vi "Config GSM Framed Timeslot.vi"(0 "VISA Resource Name":refnum<visa-resource-name>, 1 "Data (0:PN9)":T1(ring), 2 "FIX4 (0000)":i16 format="%.0b", 3 "Extended Tail Bits (3A)":i32=58 format="%.0x", 4 "User File Name (BIN_DATA)":string="BIN_DATA", 5 "error in (no error)":errorcluster {"code" format="%.0x"}, 6 "Timeslot Type (1:NORMAL)":T2(ring)=enum."NORMAL", 7 "Synch Sequence (000)":string, 8 "Status (T:ON)":bool=TRUE, 9 "Training Sequence (0970897)":string="0970897", 10 "Timeslot (0)":i16, 11 "Steal Bit (0)":i8 format="%.0x") -> (14 "VISA Resource Name Out":refnum<visa-resource-name>, 19 "error out":errorcluster {"code" format="%.0x"})   [LabVIEW 2014, in "Agilent ESG Series.lvlib"]
doc: "This VI is used configure a specified Timeslot.\nRun the Config GSM Framed.vi before running this vi.\nRun this vi multiple times to configure multiple Timeslots."
uses:
  Agilent ESG Series.lvlib
panel:
  # "ON"
  # "OFF"
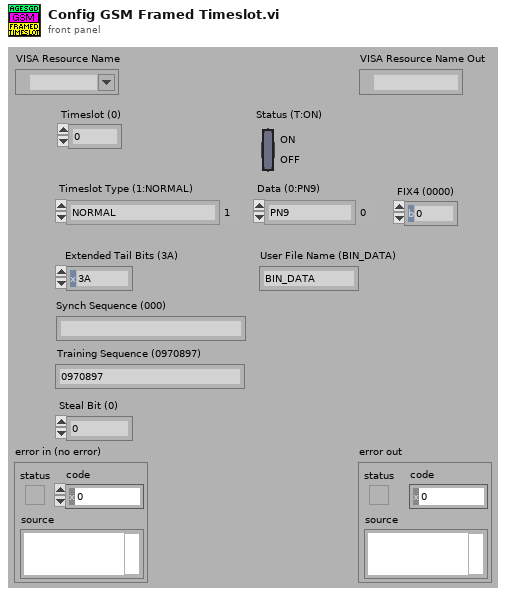
[diagram p1: front panel]
types:
  T1 = enum16{"PN9", "PN15", "FIX4", "USER FILE", "EXT", "4 1's & 4 0's", "8 1's & 8 0's", "16 1's & 16 0's", "32 1's & 32 0's", "64 1's & 64 0's"}
  T2 = enum16{"CUSTOM", "NORMAL", "FCORRECTION", "SYNC", "DUMMY", "ACCESS", "NORMAL ALL"}
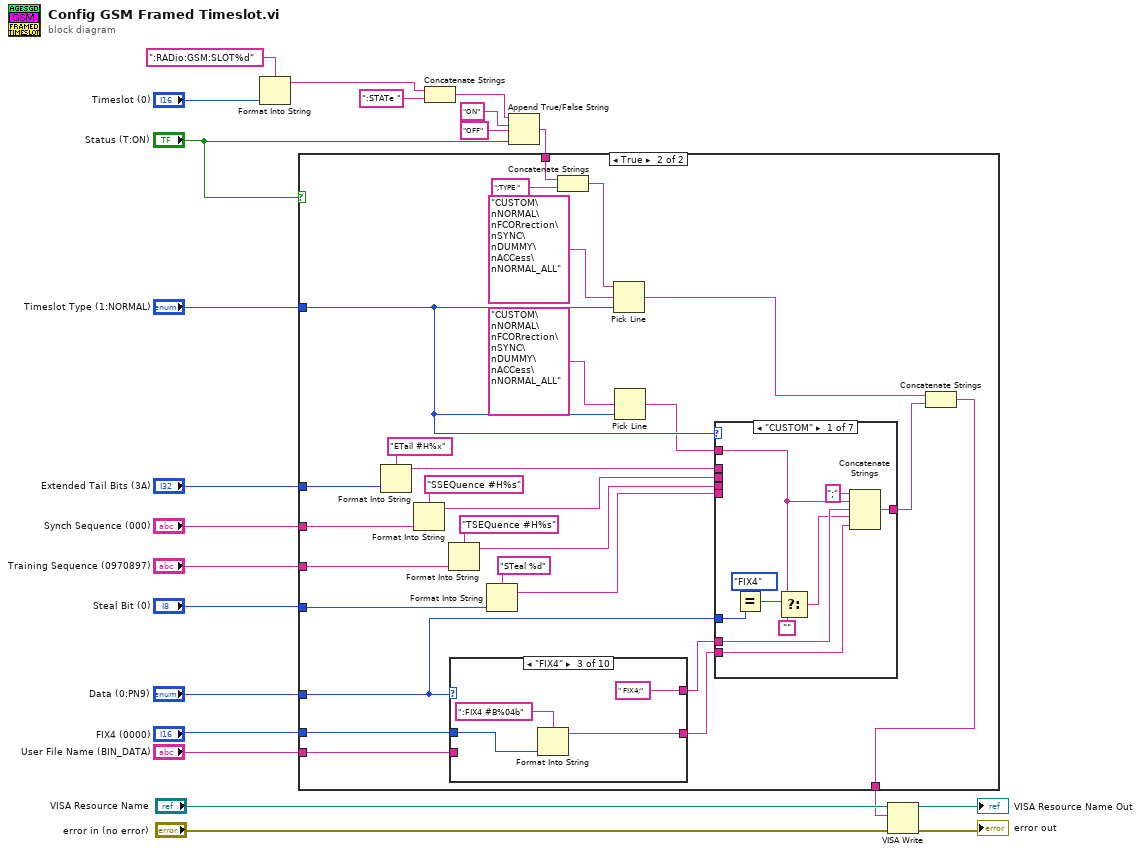
[diagram p0: block diagram]
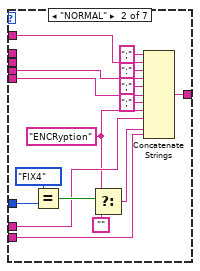
[diagram p3: hidden frame]
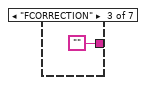
[diagram p4: hidden frame]
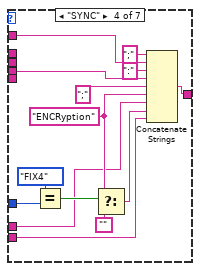
[diagram p5: hidden frame]
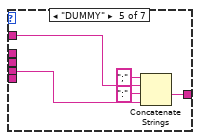
[diagram p6: hidden frame]
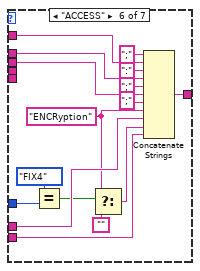
[diagram p7: hidden frame]
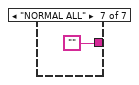
[diagram p8: hidden frame]
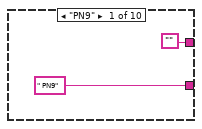
[diagram p9: hidden frame]
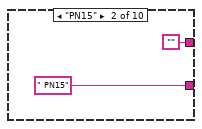
[diagram p10: hidden frame]
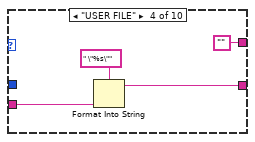
[diagram p11: hidden frame]
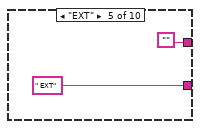
[diagram p12: hidden frame]
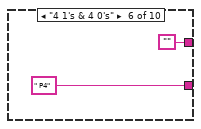
[diagram p13: hidden frame]
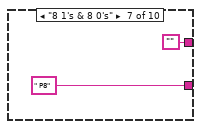
[diagram p14: hidden frame]
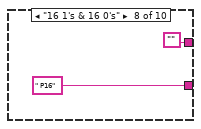
[diagram p15: hidden frame]
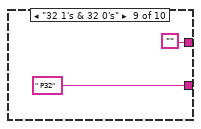
[diagram p16: hidden frame]
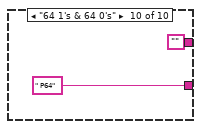
[diagram p17: hidden frame]
diagram:
  n1 = Format Into String(format string=":RADio:GSM:SLOT%d", "Timeslot (0)") -> (resulting string=w6:string)  [unwired: 2 in, 1 out]
  n2 = Concatenate Strings(w6, ":STATe ") -> (w14:string)
  n3 = Append True/False String(1:"Status (T:ON)", 2:"OFF" ("false string"), 3:"ON" ("true string"), 4:w14) -> (0:w13:string)
  n4 = case shown="True" "Status (T:ON)" {
    tunnel: [w23 w50] -> w5
    tunnel: "Timeslot Type (1:NORMAL)" -> [_ w38]
    tunnel: "FIX4 (0000)" -> [_ w48]
    tunnel: "User File Name (BIN_DATA)" -> [_ w47]
    tunnel: "Data (0:PN9)" -> [_ w24]
    tunnel: w13 -> [w23 w46]
    tunnel: "Extended Tail Bits (3A)" -> [_ w37]
    tunnel: "Synch Sequence (000)" -> [_ w33]
    tunnel: "Training Sequence (0970897)" -> [_ w30]
    tunnel: "Steal Bit (0)" -> [_ w27]
    frame False {
    }
    frame True {
      n5 = Format Into String(format string="ETail #H%x", w37) -> (resulting string=w35:string)  [unwired: 2 in, 1 out]
      n6 = Format Into String(format string="SSEQuence #H%s", w33) -> (resulting string=w32:string)  [unwired: 2 in, 1 out]
      n7 = Format Into String(format string="TSEQuence #H%s", w30) -> (resulting string=w29:string)  [unwired: 2 in, 1 out]
      n8 = case shown="\"FIX4\"" w24 {
        tunnel: w47 -> [_ _ _ w125 _ _ _ _ _ _]
        tunnel: w48 -> [_ _ w120 _ _ _ _ _ _ _]
        tunnel: [" PN9" " PN15" w119 w123 " EXT" " P4" " P8" " P16" " P32" " P64"] -> w42
        tunnel: ["" "" " FIX4;" "" "" "" "" "" "" ""] -> w39
        frame "PN9" {
        }
        frame "PN15" {
        }
        frame "FIX4" {
          n9 = Format Into String(format string=":FIX4 #B%04b", w120) -> (resulting string=w119:string)  [unwired: 2 in, 1 out]
        }
        frame "USER FILE" {
          n10 = Format Into String(format string=" \"%s\"", w125) -> (resulting string=w123:string)  [unwired: 2 in, 1 out]
        }
        frame "EXT" {
        }
        frame "4 1's & 4 0's" {
        }
        frame "8 1's & 8 0's" {
        }
        frame "16 1's & 16 0's" {
        }
        frame "32 1's & 32 0's" {
        }
        frame "64 1's & 64 0's" {
        }
      }
      n11 = Format Into String(format string="STeal %d", w27) -> (resulting string=w26:string)  [unwired: 2 in, 1 out]
      n12 = Concatenate Strings(w46, ";TYPE ") -> (w44:string)
      n13 = Pick Line(string ("")=w44, multi-line string="CUSTOM\nNORMAL\nFCORrection\nSYNC\nDUMMY\nACCess\nNORMAL_ALL", line index=w38) -> (output string=w40:string)
      n14 = Pick Line(multi-line string="CUSTOM\nNORMAL\nFCORrection\nSYNC\nDUMMY\nACCess\nNORMAL_ALL", line index=w38) -> (output string=w25:string)  [unwired: 1 in]
      n15 = case shown="\"CUSTOM\"" w38 {
        tunnel: [w59 w76 "" w80 w95 w112 ""] -> w41
        tunnel: w42 -> [w60 w69 _ w83 _ w110 _]
        tunnel: w39 -> [w58 w67 _ w84 _ w111 _]
        tunnel: w25 -> [w52 w70 _ w81 w94 w102 _]
        tunnel: w35 -> [_ _ _ _ _ w98 _]
        tunnel: w32 -> [_ _ _ _ _ w100 _]
        tunnel: w29 -> [_ w62 _ w78 w93 _ _]
        tunnel: w26 -> [_ w64 _ _ _ _ _]
        tunnel: w24 -> [w55 w74 _ w82 _ w106 _]
        frame "CUSTOM" {
          n16 = Equal?(x=T1."FIX4", y=w55) -> (x = y?=w53:bool)
          n17 = Select(t=w52, s=w53, f="") -> (s? t:f=w51:string)
          n18 = Concatenate Strings(";" ("output string"), w52, w58, w51, w60) -> (w59:string)
        }
        frame "NORMAL" {
          w66 = "ENCRyption"
          n19 = Equal?(x=T1."FIX4", y=w74) -> (x = y?=w72:bool)
          n20 = Select(t=w66, s=w72, f="") -> (s? t:f=w68:string)
          n21 = Concatenate Strings(";", w70, ":", w62, ";", w64, ";", w66, w67, w68, w69) -> (w76:string)
        }
        frame "FCORRECTION" {
        }
        frame "SYNC" {
          w89 = "ENCRyption"
          n22 = Equal?(x=T1."FIX4", y=w82) -> (x = y?=w86:bool)
          n23 = Select(t=w89, s=w86, f="") -> (s? t:f=w90:string)
          n24 = Concatenate Strings(";", w81, ":", w78, ";", w89, w84, w90, w83) -> (w80:string)
        }
        frame "DUMMY" {
          n25 = Concatenate Strings(";" ("output string"), w94, ":", w93) -> (w95:string)
        }
        frame "ACCESS" {
          w108 = "ENCRyption"
          n26 = Equal?(x=T1."FIX4", y=w106) -> (x = y?=w104:bool)
          n27 = Select(t=w108, s=w104, f="") -> (s? t:f=w109:string)
          n28 = Concatenate Strings(";", w102, ":", w98, ";", w100, ";", w108, w111, w109, w110) -> (w112:string)
        }
        frame "NORMAL ALL" {
        }
      }
      n29 = Concatenate Strings(w40, w41) -> (w50:string)
    }
  }
  n30 = VISA Write(VISA resource name="VISA Resource Name", write buffer=w5, error in (no error)="error in (no error)") -> (VISA resource name out=→"VISA Resource Name Out":refnum<visa-resource-name>, error out=→"error out":errorcluster)  [unwired: 1 out]
